vi "MCSControlPanel.vi"(4 "Register Map\nDefaults":refnum<vi>, 5 "StatusWord0x10Ref":refnum<vi>, 6 "Register Map\nRead Ref":refnum<vi>, 7 "NewRegMapReady":refnum<vi>, 8 "Last Command\nSent Ref":refnum<vi>, 9 "Stop Loop \nRef":refnum<vi>, 10 "error out":errorcluster, 11 "queue out":refnum<queue>) -> ()   [LabVIEW 2012]
panel:
  out "0x10 Status Word Readout":bool[][](array[boolean])
  in  "SYNC In \nVolt Threshold":u16
  out "word33":string
  in  "DIN In Volt \nThreshold":u16
  out "word32":string
  in  "DEMUX In Volt \nThreshold":u16
  out "word31":string
  in  "Power Mon Volt \nRef Threshold":u16
  out "word30":string
  out "wordB":string
  in  "Power Mon In 5 \nDEMUX Select":string(combo)
  in  "Power Mon In 4 \nDEMUX Select":string(combo)
  in  "Power Mon In 3 \nDEMUX Select":string(combo)
  in  "Power Mon In 2 \nDEMUX Select":string(combo)
  in  "Power Mon In 1 \nDEMUX Select":string(combo)
  in  "Power Mon In 0 \nDEMUX Select":string(combo)
  in  "Power Pulse\nReject Config":u16
  in  "Power Mon \nAcc Mode":string(combo)
  in  "Power Mon \nTest Mode":string(combo)
  in  "Power Mon Chan Enable   \n  11    10      9      8       7       6      5       4       3       2      1       0":bool[](array[boolean])
  out "word9":string
  in  "SoftDEMUX \nSelector Enable":bool
  in  "Sync Select 3B":string(combo)
  in  "Sync Select 2B":string(combo)
  in  "Sync Select 1B":string(combo)
  in  "Sync Select 0B":string(combo)
  in  "Sync Select 7":string(combo)
  in  "Sync Select 6":string(combo)
  in  "Sync Select 5":string(combo)
  in  "Sync Select 4":string(combo)
  in  "Sync Select 3A":string(combo)
  in  "Sync Select 2A":string(combo)
  in  "Sync Select 1A":string(combo)
  in  "Sync Select 0A":string(combo)
  in  "Sync Test\nMode Config":u32
  in  "Pulse Period\n(clock cycles -1)":u32
  in  "Channel DEMUX \nSelector":bool
  in  "Channel \nHold Order":bool
  in  "Channel \nTransfer Order":bool
  in  "Throttle Mode":string(combo)
  in  "Sync Test Mode Select":string(combo)
  in  "Data Input Test Mode":string(combo)
  out "Last Command Sent":string
  in  "Send Command, \nmanual entry":string
  in  "Send":bool
  in  "Reset Register Map to Defaults":bool
  in  "Sync Enable\n  2       1       0":bool[](array[boolean])
  in  "Channel Enable\n 11     10      9      8       7       6      5        4      3       2       1       0":bool[](array[boolean])
  in  "Reset Profile Accumulator  \n  11     10     9      8       7       6      5       4       3      2       1       0":bool[](array[boolean])
  in  "Counts Per Bin":u16
  in  "User Reset":bool
  in  "Number of Bins":u16
  in  "Profiles Per Histogram":u16
  in  "Time Reset":bool
  in  "Relative Time Step":u32
  in  "Demux Channel Enable\n  3       2       1      0":bool[](array[boolean])
  out "word0":string
  out "word1":string
  out "word2":string
  out "word3":string
  out "word4":string
  out "word5":string
  out "word6":string
  out "word7":string
  out "word8":string
  in  "DIN Polarity \n  7      6        5      4       3       2      1       0":bool[](array[boolean])
  in  "DIN Demux Polarity\n  3       2       1      0":bool[](array[boolean])
  in  "Sync Input Polarity\n  2       1       0":bool[](array[boolean])
  in  "PIN0 Pulse \nDurration Ave 2^N":u16
  out "wordA":string
  in  "PIN1 Pulse \nDurration Ave 2^N":u16
  in  "PIN2 Pulse \nDurration Ave 2^N":u16
  in  "PIN3 Pulse \nDurration Ave 2^N":u16
  in  "PIN4 Pulse \nDurration Ave 2^N":u16
  in  "PIN5 Pulse \nDurration Ave 2^N":u16
  # "word00"
  # "word30"
  # "valid range (0-65535)"
  # "word01"
  # "word02"
  # "word03"
  # "word04"
  # "word31"
  # "valid range (2-4096)"
  # "valid range (2-4096)"
  # "valid range (1-32,768)"
  # "valid range (0-65535)"
  # "word32"
  # "word05"
  # "valid range (0-65535)"
  # "word33"
  # "word06"
  # "valid range (0-65535)"
  # "valid range (0-256)"
  # "valid range (0-64)"
  # "word07"
  # "word08"
  # "word09"
  # "valid range (0-33,554,432)"
  # "valid range (0-256)"
  # "word0A"
  # "word0B"
  # "N=valid range (0-15)"
  # "N=valid range (0-15)"
  # "N=valid range (0-15)"
  # "N=valid range (0-15)"
  # "N=valid range (0-15)"
  # "N=valid range (0-15)"
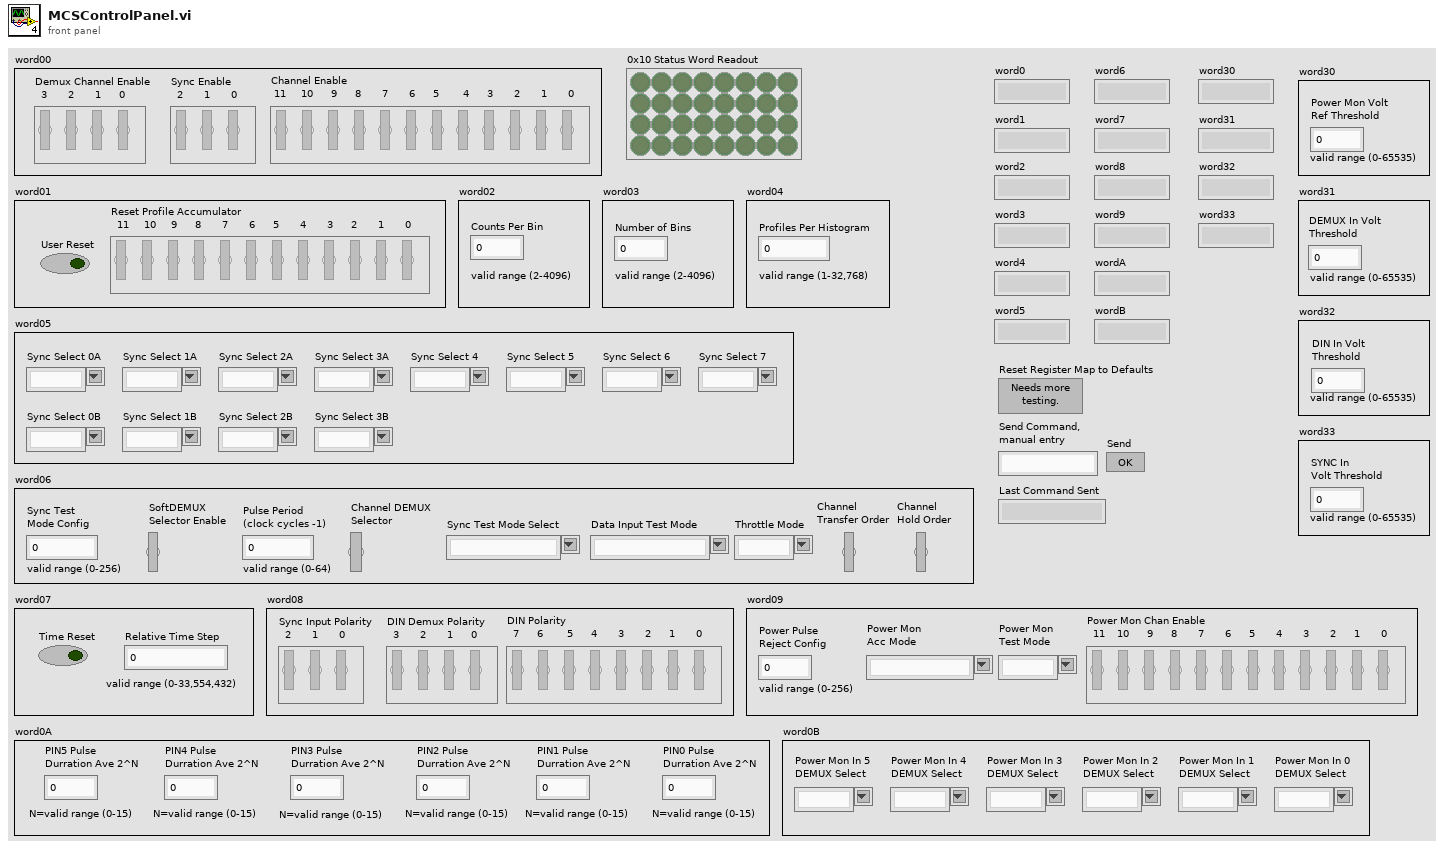
[diagram p1: front panel]
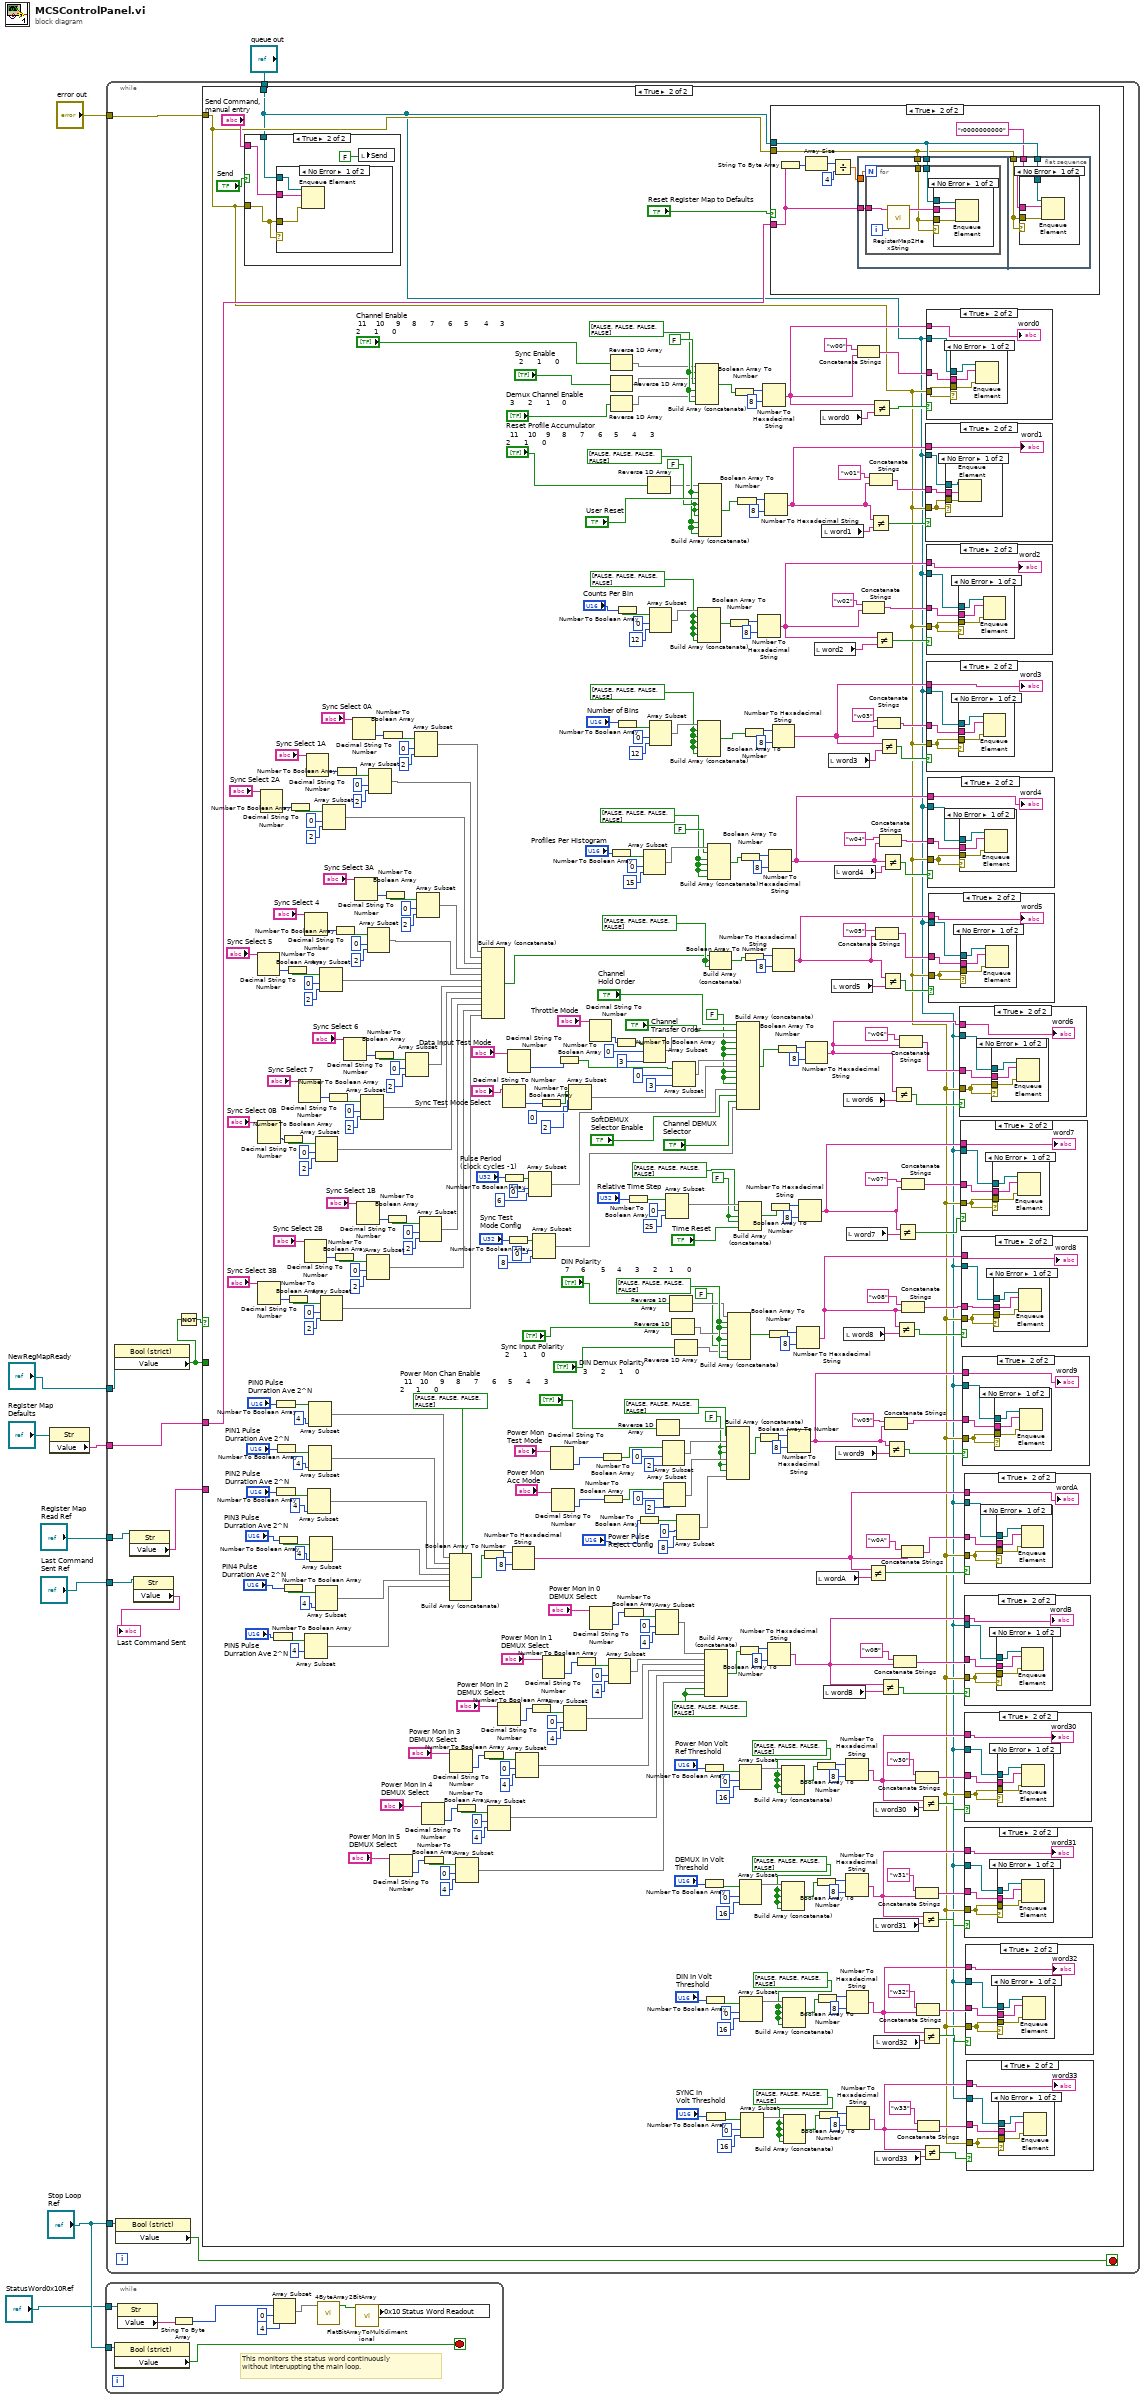
[diagram p0: block diagram]
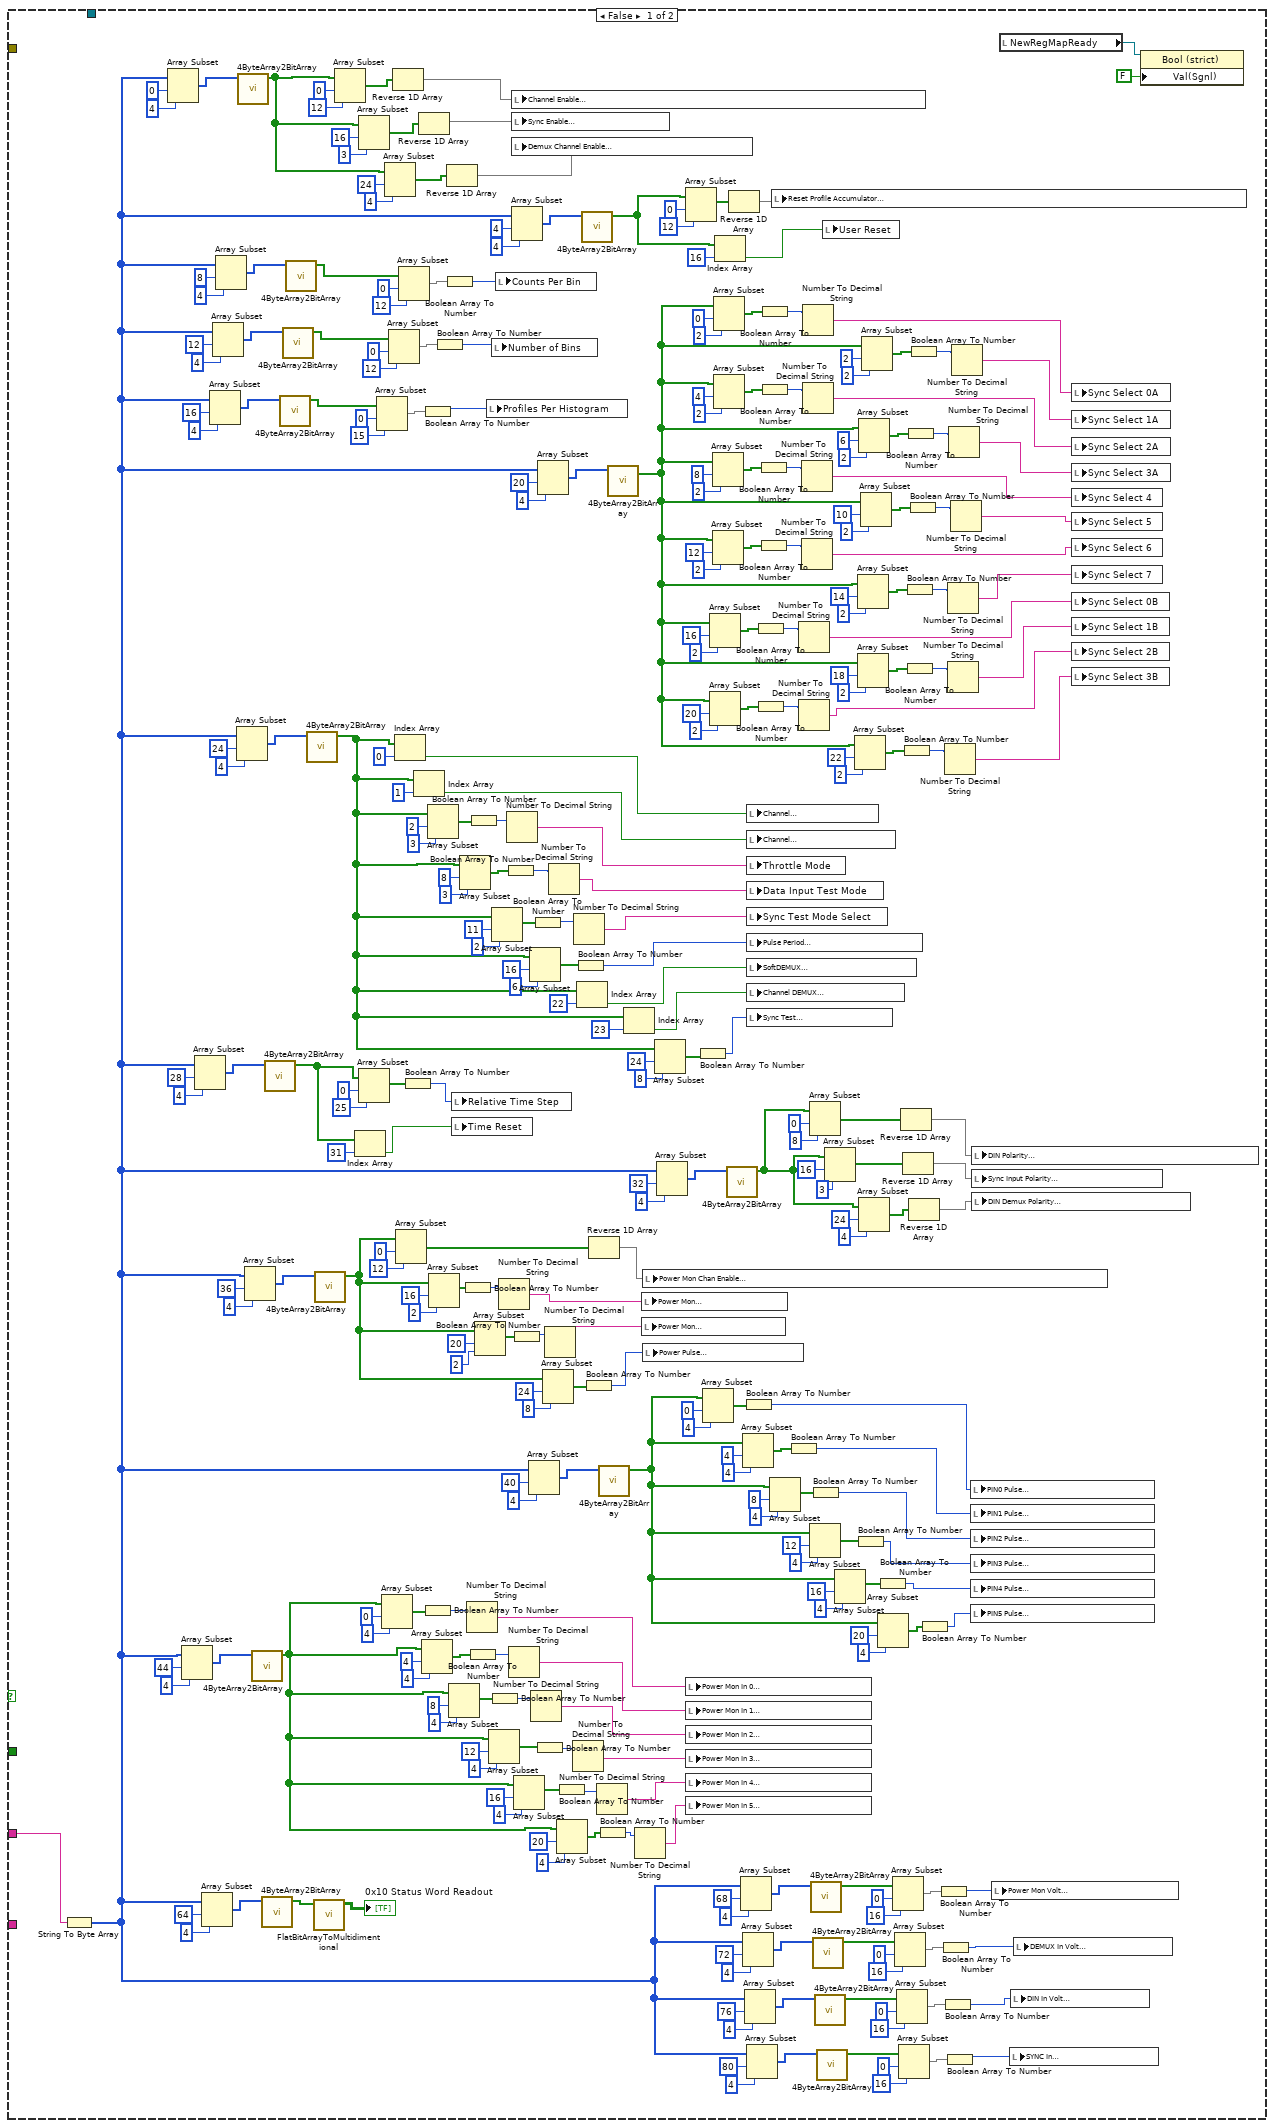
[diagram p2: hidden frame]
diagram:
  n1 = property class="Str"(reference="Register Map\nDefaults") -> ("Value"=w3:string)  [unwired: 1 in, 2 out]
  n2 = while {
    tunnel: "Stop Loop \nRef" -> [w14]
    tunnel: "StatusWord0x10Ref" -> [w11]
    stop <- w13 stop-if-true
    # "This monitors the status word continuously\nwithout interuppting the main loop."
    n3 = property class="Bool (strict)"(reference=w14) -> ("Value"=w13:bool)  [unwired: 1 in, 2 out]
    n4 = property class="Str"(reference=w11) -> ("Value"=w12:string)  [unwired: 1 in, 2 out]
    n5 = String To Byte Array(string=w12) -> (unsigned byte array=w17:u8[])
    n6 = Array Subset(array=w17, index=0, length=4) -> (w16:u8[])
    n7 = call "4ByteArray2BitArray.vi"("array"=w16) -> ("Array"=w15:bool[])  [unwired: 10 in]
    n8 = call "FlatBitArrayToMultidimentional.vi"("Array in"=w15) -> ("Array out"=w10:bool[][])  [unwired: 10 in]
    n9 = local write "0x10 Status Word Readout"(w10) -> ()
  }
  n10 = while {
    tunnel: "queue out" -> [w31]
    tunnel: "error out" -> [w30]
    tunnel: "Stop Loop \nRef" -> [w29]
    tunnel: "Last Command\nSent Ref" -> [w25]
    tunnel: "Register Map\nRead Ref" -> [w26]
    tunnel: w3 -> [w22]
    tunnel: "NewRegMapReady" -> [w23]
    stop <- w28 stop-if-true
    n11 = property class="Bool (strict)"(reference=w23) -> ("Value"=w20:bool)  [unwired: 1 in, 2 out]
    n12 = property class="Bool (strict)"(reference=w29) -> ("Value"=w28:bool)  [unwired: 1 in, 2 out]
    n13 = property class="Str"(reference=w26) -> ("Value"=w24:string)  [unwired: 1 in, 2 out]
    n14 = property class="Str"(reference=w25) -> ("Value"=→"Last Command Sent":string)  [unwired: 1 in, 2 out]
    n15 = Not(x=w20) -> (.not. x?=w21:bool)
    n16 = case shown="True" w21 {
      tunnel: w31 -> [_ w338]
      tunnel: w30 -> [_ w339]
      tunnel: w24 -> [_ _]
      tunnel: w22 -> [w54 w514]
      tunnel: w20 -> [_ _]
      frame False {
        n17 = String To Byte Array(string=w54) -> (unsigned byte array=w51:u8[])
        n18 = Array Subset(array=w51, index=0, length=4) -> (w300:u8[])
        n19 = Array Subset(array=w51, index=44, length=4) -> (w118:u8[])
        n20 = Array Subset(array=w51, index=28, length=4) -> (w306:u8[])
        n21 = Array Subset(array=w51, index=64, length=4) -> (w50:u8[])
        n22 = Array Subset(array=w51, index=16, length=4) -> (w315:u8[])
        n23 = Array Subset(array=w51, index=12, length=4) -> (w318:u8[])
        n24 = Array Subset(array=w51, index=8, length=4) -> (w321:u8[])
        n25 = Array Subset(array=w51, index=24, length=4) -> (w309:u8[])
        n26 = call "4ByteArray2BitArray.vi"("array"=w300) -> ("Array"=w146:bool[])  [unwired: 10 in]
        n27 = Array Subset(array=w51, index=36, length=4) -> (w140:u8[])
        n28 = call "4ByteArray2BitArray.vi"("array"=w118) -> ("Array"=w99:bool[])  [unwired: 10 in]
        n29 = call "4ByteArray2BitArray.vi"("array"=w50) -> ("Array"=w33:bool[])  [unwired: 10 in]
        n30 = call "4ByteArray2BitArray.vi"("array"=w306) -> ("Array"=w265:bool[])  [unwired: 10 in]
        n31 = call "4ByteArray2BitArray.vi"("array"=w315) -> ("Array"=w167:bool[])  [unwired: 10 in]
        n32 = call "4ByteArray2BitArray.vi"("array"=w318) -> ("Array"=w162:bool[])  [unwired: 10 in]
        n33 = call "4ByteArray2BitArray.vi"("array"=w321) -> ("Array"=w157:bool[])  [unwired: 10 in]
        n34 = call "4ByteArray2BitArray.vi"("array"=w309) -> ("Array"=w145:bool[])  [unwired: 10 in]
        n35 = call "FlatBitArrayToMultidimentional.vi"("Array in"=w33) -> ("Array out"=→"0x10 Status Word Readout":bool[][])  [unwired: 10 in]
        n36 = call "4ByteArray2BitArray.vi"("array"=w140) -> ("Array"=w127:bool[])  [unwired: 10 in]
        n37 = Array Subset(array=w146, index=0, length=12) -> (w48:bool[])
        n38 = Index Array(array=w265, index=31) -> (element=w263:bool)
        n39 = Array Subset(array=w146, index=16, length=3) -> (w46:bool[])
        n40 = Array Subset(array=w265, index=0, length=25) -> (w261:bool[])
        n41 = Array Subset(array=w167, index=0, length=15) -> (w168:bool[])
        n42 = Array Subset(array=w99, index=0, length=4) -> (w104:bool[])
        n43 = Array Subset(array=w146, index=24, length=4) -> (w44:bool[])
        n44 = Array Subset(array=w162, index=0, length=12) -> (w163:bool[])
        n45 = Reverse 1D Array(array=w48) -> (reversed array=w49:bool[])
        n46 = Index Array(array=w145, index=0) -> (element=w243:bool)
        n47 = Array Subset(array=w127, index=0, length=12) -> (w34:bool[])
        n48 = Array Subset(array=w157, index=0, length=12) -> (w158:bool[])
        n49 = Boolean Array To Number(Boolean array=w261) -> (number=w262:u32)
        n50 = Index Array(array=w145, index=1) -> (element=w242:bool)
        n51 = Reverse 1D Array(array=w46) -> (reversed array=w47:bool[])
        n52 = Array Subset(array=w99, index=4, length=4) -> (w105:bool[])
        n53 = Boolean Array To Number(Boolean array=w168) -> (number=w166:u32)
        n54 = Boolean Array To Number(Boolean array=w104) -> (number=w98:u32)
        n55 = Array Subset(array=w145, index=2, length=3) -> (w249:bool[])
        n56 = Array Subset(array=w127, index=16, length=2) -> (w136:bool[])
        n57 = Boolean Array To Number(Boolean array=w163) -> (number=w161:u32)
        n58 = Boolean Array To Number(Boolean array=w158) -> (number=w156:u32)
        n59 = Reverse 1D Array(array=w44) -> (reversed array=w45:bool[])
        n60 = Array Subset(array=w99, index=8, length=4) -> (w103:bool[])
        n61 = local write "Relative Time Step"(w262) -> ()
        n62 = local write "Time Reset"(w263) -> ()
        n63 = Array Subset(array=w145, index=8, length=3) -> (w250:bool[])
        n64 = Boolean Array To Number(Boolean array=w136) -> (number=w135:u32)
        n65 = Number To Decimal String(number=w98) -> (decimal integer string=w87:string)  [unwired: 1 in]
        n66 = Boolean Array To Number(Boolean array=w105) -> (number=w97:u32)
        n67 = Boolean Array To Number(Boolean array=w249) -> (number=w241:u32)
        n68 = Array Subset(array=w127, index=20, length=2) -> (w132:bool[])
        n69 = local write "Profiles Per Histogram"(w166) -> ()
        n70 = Array Subset(array=w99, index=12, length=4) -> (w102:bool[])
        n71 = Boolean Array To Number(Boolean array=w103) -> (number=w96:u32)
        n72 = local write "Number of Bins"(w161) -> ()
        n73 = Array Subset(array=w145, index=11, length=2) -> (w248:bool[])
        n74 = local write "Counts Per Bin"(w156) -> ()
        n75 = Number To Decimal String(number=w135) -> (decimal integer string=w134:string)  [unwired: 1 in]
        n76 = Boolean Array To Number(Boolean array=w250) -> (number=w239:u32)
        n77 = Number To Decimal String(number=w241) -> (decimal integer string=w240:string)  [unwired: 1 in]
        n78 = Number To Decimal String(number=w97) -> (decimal integer string=w88:string)  [unwired: 1 in]
        n79 = local write "Channel Enable\n 11     10      9      8       7       6      5        4      3       2       1       0"(w49) -> ()
        n80 = local write "Sync Enable\n  2       1       0"(w47) -> ()
        n81 = local write "Demux Channel Enable\n  3       2       1      0"(w45) -> ()
        n82 = Array Subset(array=w51, index=4, length=4) -> (w324:u8[])
        n83 = Boolean Array To Number(Boolean array=w132) -> (number=w131:u32)
        n84 = Array Subset(array=w99, index=16, length=4) -> (w101:bool[])
        n85 = Array Subset(array=w51, index=40, length=4) -> (w327:u8[])
        n86 = Array Subset(array=w145, index=16, length=6) -> (w247:bool[])
        n87 = Number To Decimal String(number=w96) -> (decimal integer string=w89:string)  [unwired: 1 in]
        n88 = Boolean Array To Number(Boolean array=w248) -> (number=w237:u32)
        n89 = Boolean Array To Number(Boolean array=w102) -> (number=w94:u32)
        n90 = Array Subset(array=w51, index=20, length=4) -> (w312:u8[])
        n91 = Array Subset(array=w127, index=24, length=8) -> (w128:bool[])
        n92 = Number To Decimal String(number=w131) -> (decimal integer string=w130:string)  [unwired: 1 in]
        n93 = Number To Decimal String(number=w239) -> (decimal integer string=w238:string)  [unwired: 1 in]
        n94 = Boolean Array To Number(Boolean array=w101) -> (number=w95:u32)
        n95 = Array Subset(array=w99, index=20, length=4) -> (w100:bool[])
        n96 = Number To Decimal String(number=w94) -> (decimal integer string=w90:string)  [unwired: 1 in]
        n97 = Number To Decimal String(number=w237) -> (decimal integer string=w236:string)  [unwired: 1 in]
        n98 = Boolean Array To Number(Boolean array=w247) -> (number=w233:u32)
        n99 = Index Array(array=w145, index=22) -> (element=w143:bool)
        n100 = call "4ByteArray2BitArray.vi"("array"=w324) -> ("Array"=w152:bool[])  [unwired: 10 in]
        n101 = Boolean Array To Number(Boolean array=w128) -> (number=w126:u32)
        n102 = Reverse 1D Array(array=w34) -> (reversed array=w35:bool[])
        n103 = Number To Decimal String(number=w95) -> (decimal integer string=w91:string)  [unwired: 1 in]
        n104 = Boolean Array To Number(Boolean array=w100) -> (number=w93:u32)
        n105 = call "4ByteArray2BitArray.vi"("array"=w327) -> ("Array"=w287:bool[])  [unwired: 10 in]
        n106 = call "4ByteArray2BitArray.vi"("array"=w312) -> ("Array"=w183:bool[])  [unwired: 10 in]
        n107 = Index Array(array=w145, index=23) -> (element=w234:bool)
        n108 = Number To Decimal String(number=w93) -> (decimal integer string=w92:string)  [unwired: 1 in]
        n109 = local write "Power Mon \nTest Mode"(w134) -> ()
        n110 = local write "Power Mon \nAcc Mode"(w130) -> ()
        n111 = local write "Power Mon Chan Enable   \n  11    10      9      8       7       6      5       4       3       2      1       0"(w35) -> ()
        n112 = local write "Power Pulse\nReject Config"(w126) -> ()
        n113 = Array Subset(array=w145, index=24, length=8) -> (w246:bool[])
        n114 = Array Subset(array=w51, index=32, length=4) -> (w303:u8[])
        n115 = Array Subset(array=w152, index=0, length=12) -> (w42:bool[])
        n116 = local write "Power Mon In 0 \nDEMUX Select"(w87) -> ()
        n117 = local write "Power Mon In 1 \nDEMUX Select"(w88) -> ()
        n118 = local write "Power Mon In 2 \nDEMUX Select"(w89) -> ()
        n119 = local write "Power Mon In 3 \nDEMUX Select"(w90) -> ()
        n120 = local write "Power Mon In 4 \nDEMUX Select"(w91) -> ()
        n121 = local write "Power Mon In 5 \nDEMUX Select"(w92) -> ()
        n122 = Boolean Array To Number(Boolean array=w246) -> (number=w232:u32)
        n123 = Array Subset(array=w287, index=0, length=4) -> (w284:bool[])
        n124 = Array Subset(array=w183, index=16, length=2) -> (w197:bool[])
        n125 = Array Subset(array=w183, index=20, length=2) -> (w189:bool[])
        n126 = Array Subset(array=w183, index=8, length=2) -> (w213:bool[])
        n127 = Array Subset(array=w183, index=12, length=2) -> (w205:bool[])
        n128 = Array Subset(array=w183, index=0, length=2) -> (w229:bool[])
        n129 = Array Subset(array=w183, index=4, length=2) -> (w221:bool[])
        n130 = Index Array(array=w152, index=16) -> (element=w151:bool)
        n131 = call "4ByteArray2BitArray.vi"("array"=w303) -> ("Array"=w268:bool[])  [unwired: 10 in]
        n132 = Reverse 1D Array(array=w42) -> (reversed array=w43:bool[])
        n133 = Array Subset(array=w51, index=68, length=4) -> (w84:u8[])
        n134 = Array Subset(array=w287, index=4, length=4) -> (w286:bool[])
        n135 = Array Subset(array=w51, index=72, length=4) -> (w77:u8[])
        n136 = Boolean Array To Number(Boolean array=w284) -> (number=w283:u32)
        n137 = Array Subset(array=w51, index=76, length=4) -> (w70:u8[])
        n138 = local write "Channel \nHold Order"(w243) -> ()
        n139 = local write "Channel \nTransfer Order"(w242) -> ()
        n140 = local write "Throttle Mode"(w240) -> ()
        n141 = local write "Data Input Test Mode"(w238) -> ()
        n142 = local write "Sync Test Mode Select"(w236) -> ()
        n143 = local write "Pulse Period\n(clock cycles -1)"(w233) -> ()
        n144 = local write "SoftDEMUX \nSelector Enable"(w143) -> ()
        n145 = local write "Channel DEMUX \nSelector"(w234) -> ()
        n146 = local write "Sync Test\nMode Config"(w232) -> ()
        n147 = Array Subset(array=w51, index=80, length=4) -> (w63:u8[])
        n148 = Boolean Array To Number(Boolean array=w197) -> (number=w196:u32)
        n149 = Boolean Array To Number(Boolean array=w189) -> (number=w188:u32)
        n150 = Boolean Array To Number(Boolean array=w213) -> (number=w212:u32)
        n151 = Boolean Array To Number(Boolean array=w205) -> (number=w204:u32)
        n152 = Boolean Array To Number(Boolean array=w229) -> (number=w228:u32)
        n153 = Boolean Array To Number(Boolean array=w221) -> (number=w220:u32)
        n154 = Array Subset(array=w287, index=8, length=4) -> (w281:bool[])
        n155 = local write "Reset Profile Accumulator  \n  11     10     9      8       7       6      5       4       3      2       1       0"(w43) -> ()
        n156 = Boolean Array To Number(Boolean array=w286) -> (number=w285:u32)
        n157 = Number To Decimal String(number=w196) -> (decimal integer string=w174:string)  [unwired: 1 in]
        n158 = Number To Decimal String(number=w188) -> (decimal integer string=w172:string)  [unwired: 1 in]
        n159 = Number To Decimal String(number=w212) -> (decimal integer string=w178:string)  [unwired: 1 in]
        n160 = Number To Decimal String(number=w204) -> (decimal integer string=w176:string)  [unwired: 1 in]
        n161 = Number To Decimal String(number=w228) -> (decimal integer string=w182:string)  [unwired: 1 in]
        n162 = Number To Decimal String(number=w220) -> (decimal integer string=w180:string)  [unwired: 1 in]
        n163 = Array Subset(array=w268, index=0, length=8) -> (w36:bool[])
        n164 = Array Subset(array=w287, index=12, length=4) -> (w280:bool[])
        n165 = Boolean Array To Number(Boolean array=w281) -> (number=w282:u32)
        n166 = call "4ByteArray2BitArray.vi"("array"=w84) -> ("Array"=w80:bool[])  [unwired: 10 in]
        n167 = call "4ByteArray2BitArray.vi"("array"=w77) -> ("Array"=w73:bool[])  [unwired: 10 in]
        n168 = call "4ByteArray2BitArray.vi"("array"=w70) -> ("Array"=w66:bool[])  [unwired: 10 in]
        n169 = call "4ByteArray2BitArray.vi"("array"=w63) -> ("Array"=w59:bool[])  [unwired: 10 in]
        n170 = local write "User Reset"(w151) -> ()
        n171 = Array Subset(array=w268, index=16, length=3) -> (w37:bool[])
        n172 = Array Subset(array=w287, index=16, length=4) -> (w279:bool[])
        n173 = Array Subset(array=w183, index=22, length=2) -> (w185:bool[])
        n174 = Boolean Array To Number(Boolean array=w280) -> (number=w275:u32)
        n175 = Array Subset(array=w183, index=14, length=2) -> (w201:bool[])
        n176 = Array Subset(array=w183, index=18, length=2) -> (w193:bool[])
        n177 = Array Subset(array=w183, index=6, length=2) -> (w217:bool[])
        n178 = Array Subset(array=w268, index=24, length=4) -> (w38:bool[])
        n179 = Array Subset(array=w183, index=10, length=2) -> (w209:bool[])
        n180 = Array Subset(array=w183, index=2, length=2) -> (w225:bool[])
        n181 = Boolean Array To Number(Boolean array=w279) -> (number=w276:u32)
        n182 = Array Subset(array=w287, index=20, length=4) -> (w278:bool[])
        n183 = Array Subset(array=w80, index=0, length=16) -> (w81:bool[])
        n184 = Array Subset(array=w73, index=0, length=16) -> (w74:bool[])
        n185 = Array Subset(array=w66, index=0, length=16) -> (w67:bool[])
        n186 = Array Subset(array=w59, index=0, length=16) -> (w60:bool[])
        n187 = Reverse 1D Array(array=w36) -> (reversed array=w41:bool[])
        n188 = Boolean Array To Number(Boolean array=w185) -> (number=w184:u32)
        n189 = Reverse 1D Array(array=w37) -> (reversed array=w40:bool[])
        n190 = Boolean Array To Number(Boolean array=w201) -> (number=w200:u32)
        n191 = Boolean Array To Number(Boolean array=w193) -> (number=w192:u32)
        n192 = Boolean Array To Number(Boolean array=w217) -> (number=w216:u32)
        n193 = Boolean Array To Number(Boolean array=w209) -> (number=w208:u32)
        n194 = Boolean Array To Number(Boolean array=w225) -> (number=w224:u32)
        n195 = Reverse 1D Array(array=w38) -> (reversed array=w39:bool[])
        n196 = Boolean Array To Number(Boolean array=w278) -> (number=w277:u32)
        n197 = Boolean Array To Number(Boolean array=w81) -> (number=w58:u32)
        n198 = Boolean Array To Number(Boolean array=w74) -> (number=w57:u32)
        n199 = Boolean Array To Number(Boolean array=w67) -> (number=w56:u32)
        n200 = Number To Decimal String(number=w184) -> (decimal integer string=w171:string)  [unwired: 1 in]
        n201 = Boolean Array To Number(Boolean array=w60) -> (number=w55:u32)
        n202 = Number To Decimal String(number=w200) -> (decimal integer string=w175:string)  [unwired: 1 in]
        n203 = Number To Decimal String(number=w192) -> (decimal integer string=w173:string)  [unwired: 1 in]
        n204 = Number To Decimal String(number=w216) -> (decimal integer string=w179:string)  [unwired: 1 in]
        n205 = Number To Decimal String(number=w208) -> (decimal integer string=w177:string)  [unwired: 1 in]
        n206 = Number To Decimal String(number=w224) -> (decimal integer string=w181:string)  [unwired: 1 in]
        n207 = local write "PIN0 Pulse \nDurration Ave 2^N"(w283) -> ()
        n208 = local write "PIN1 Pulse \nDurration Ave 2^N"(w285) -> ()
        n209 = local write "PIN2 Pulse \nDurration Ave 2^N"(w282) -> ()
        n210 = local write "PIN3 Pulse \nDurration Ave 2^N"(w275) -> ()
        n211 = local write "PIN4 Pulse \nDurration Ave 2^N"(w276) -> ()
        n212 = local write "PIN5 Pulse \nDurration Ave 2^N"(w277) -> ()
        n213 = local write "DIN Polarity \n  7      6        5      4       3       2      1       0"(w41) -> ()
        n214 = local write "Sync Input Polarity\n  2       1       0"(w40) -> ()
        n215 = local write "DIN Demux Polarity\n  3       2       1      0"(w39) -> ()
        n216 = local write "Power Mon Volt \nRef Threshold"(w58) -> ()
        n217 = local read "NewRegMapReady"() -> (w122:refnum<vi>)
        n218 = local write "SYNC In \nVolt Threshold"(w55) -> ()
        n219 = local write "DIN In Volt \nThreshold"(w56) -> ()
        n220 = local write "DEMUX In Volt \nThreshold"(w57) -> ()
        n221 = local write "Sync Select 0A"(w182) -> ()
        n222 = local write "Sync Select 1A"(w181) -> ()
        n223 = local write "Sync Select 2A"(w180) -> ()
        n224 = local write "Sync Select 3A"(w179) -> ()
        n225 = local write "Sync Select 4"(w178) -> ()
        n226 = local write "Sync Select 5"(w177) -> ()
        n227 = local write "Sync Select 6"(w176) -> ()
        n228 = local write "Sync Select 7"(w175) -> ()
        n229 = local write "Sync Select 0B"(w174) -> ()
        n230 = local write "Sync Select 1B"(w173) -> ()
        n231 = local write "Sync Select 2B"(w172) -> ()
        n232 = local write "Sync Select 3B"(w171) -> ()
        n233 = property class="Bool (strict)"(reference=w122, "Val(Sgnl)"=FALSE ("Value (Signaling)")) -> ()  [unwired: 1 in, 2 out]
      }
      frame True {
        w340 = bool[] [FALSE, FALSE, FALSE, FALSE] ("appended array")
        w354 = bool[] [FALSE, FALSE, FALSE, FALSE] ("appended array")
        w368 = bool[] [FALSE, FALSE, FALSE, FALSE] ("appended array")
        w382 = bool[] [FALSE, FALSE, FALSE, FALSE] ("appended array")
        w443 = bool[] [FALSE, FALSE, FALSE, FALSE] ("appended array")
        w333 = FALSE ("Read Register")
        w666 = bool[] [FALSE, FALSE, FALSE, FALSE] ("appended array")
        w690 = bool[] [FALSE, FALSE, FALSE, FALSE] ("appended array")
        w692 = FALSE ("Read Register")
        w625 = FALSE ("Read Register")
        w697 = bool[] [FALSE, FALSE, FALSE, FALSE] ("appended array")
        w546 = bool[] [FALSE, FALSE, FALSE, FALSE] ("appended array")
        w695 = bool[] [FALSE, FALSE, FALSE, FALSE] ("appended array")
        w696 = bool[] [FALSE, FALSE, FALSE, FALSE] ("appended array")
        w710 = FALSE ("Read Register")
        w709 = bool[] [FALSE, FALSE, FALSE, FALSE] ("appended array")
        w712 = bool[] [FALSE, FALSE, FALSE, FALSE] ("appended array")
        n234 = case shown="True" "Send" {
          tunnel: "Send Command, \nmanual entry" -> [_ w869]
          tunnel: w338 -> [_ w868]
          tunnel: w339 -> [_ w866]
          frame False {
          }
          frame True {
            n235 = case shown="No Error" w866 {
              tunnel: w869 -> [w872 _]
              tunnel: w866 -> [w871 _]
              tunnel: w868 -> [w870 _]
              frame No Error {
                n236 = Enqueue Element(queue=w870, element=w872, error in (no error)=w871) -> ()  [unwired: 1 in, 3 out]
              }
              frame Error {
              }
            }
            n237 = local write "Send"(FALSE ("Send")) -> ()
          }
        }
        n238 = Decimal String To Number(string="Sync Select 5") -> (number=w590:i32)  [unwired: 2 in, 1 out]
        n239 = Decimal String To Number(string="Sync Select 0B") -> (number=w575:i32)  [unwired: 2 in, 1 out]
        n240 = Decimal String To Number(string="Sync Select 3B") -> (number=w560:i32)  [unwired: 2 in, 1 out]
        n241 = Decimal String To Number(string="Sync Select 2A") -> (number=w605:i32)  [unwired: 2 in, 1 out]
        n242 = Number To Boolean Array(number="PIN5 Pulse \nDurration Ave 2^N") -> (Boolean array=w682:bool[])
        n243 = Number To Boolean Array(number="PIN0 Pulse \nDurration Ave 2^N") -> (Boolean array=w688:bool[])
        n244 = Number To Boolean Array(number="PIN2 Pulse \nDurration Ave 2^N") -> (Boolean array=w678:bool[])
        n245 = Number To Boolean Array(number="PIN1 Pulse \nDurration Ave 2^N") -> (Boolean array=w686:bool[])
        n246 = Number To Boolean Array(number="PIN3 Pulse \nDurration Ave 2^N") -> (Boolean array=w680:bool[])
        n247 = Number To Boolean Array(number=w575) -> (Boolean array=w577:bool[])
        n248 = Number To Boolean Array(number="PIN4 Pulse \nDurration Ave 2^N") -> (Boolean array=w684:bool[])
        n249 = Number To Boolean Array(number=w590) -> (Boolean array=w592:bool[])
        n250 = Number To Boolean Array(number=w560) -> (Boolean array=w562:bool[])
        n251 = Number To Boolean Array(number=w605) -> (Boolean array=w607:bool[])
        n252 = Decimal String To Number(string="Sync Select 7") -> (number=w580:i32)  [unwired: 2 in, 1 out]
        n253 = Decimal String To Number(string="Sync Select 2B") -> (number=w565:i32)  [unwired: 2 in, 1 out]
        n254 = Decimal String To Number(string="Sync Select 4") -> (number=w595:i32)  [unwired: 2 in, 1 out]
        n255 = Array Subset(array=w682, length=4) -> (w667:bool[])  [unwired: 1 in]
        n256 = Decimal String To Number(string="Sync Select 1A") -> (number=w610:i32)  [unwired: 2 in, 1 out]
        n257 = Array Subset(array=w678, length=4) -> (w670:bool[])  [unwired: 1 in]
        n258 = Array Subset(array=w688, length=4) -> (w672:bool[])  [unwired: 1 in]
        n259 = Array Subset(array=w686, length=4) -> (w671:bool[])  [unwired: 1 in]
        n260 = Array Subset(array=w680, length=4) -> (w669:bool[])  [unwired: 1 in]
        n261 = Array Subset(array=w577, index=0, length=2) -> (w550:bool[])
        n262 = Array Subset(array=w684, length=4) -> (w668:bool[])  [unwired: 1 in]
        n263 = Array Subset(array=w592, index=0, length=2) -> (w554:bool[])
        n264 = Array Subset(array=w562, index=0, length=2) -> (w553:bool[])
        n265 = Array Subset(array=w607, index=0, length=2) -> (w557:bool[])
        n266 = Number To Boolean Array(number=w580) -> (Boolean array=w582:bool[])
        n267 = Number To Boolean Array(number=w565) -> (Boolean array=w567:bool[])
        n268 = Number To Boolean Array(number=w595) -> (Boolean array=w597:bool[])
        n269 = Number To Boolean Array(number=w610) -> (Boolean array=w612:bool[])
        n270 = Decimal String To Number(string="Sync Select 6") -> (number=w585:i32)  [unwired: 2 in, 1 out]
        n271 = Decimal String To Number(string="Sync Select 0A") -> (number=w615:i32)  [unwired: 2 in, 1 out]
        n272 = Decimal String To Number(string="Sync Select 3A") -> (number=w600:i32)  [unwired: 2 in, 1 out]
        n273 = Decimal String To Number(string="Sync Select 1B") -> (number=w570:i32)  [unwired: 2 in, 1 out]
        n274 = Array Subset(array=w582, index=0, length=2) -> (w549:bool[])
        n275 = Array Subset(array=w567, index=0, length=2) -> (w552:bool[])
        n276 = Array Subset(array=w597, index=0, length=2) -> (w555:bool[])
        n277 = Array Subset(array=w612, index=0, length=2) -> (w558:bool[])
        n278 = Number To Boolean Array(number=w585) -> (Boolean array=w587:bool[])
        n279 = Number To Boolean Array(number=w615) -> (Boolean array=w617:bool[])
        n280 = Number To Boolean Array(number=w600) -> (Boolean array=w602:bool[])
        n281 = Number To Boolean Array(number=w570) -> (Boolean array=w572:bool[])
        n282 = Decimal String To Number(string="Power Mon In 5 \nDEMUX Select") -> (number=w446:i32)  [unwired: 2 in, 1 out]
        n283 = Array Subset(array=w587, index=0, length=2) -> (w548:bool[])
        n284 = Array Subset(array=w617, index=0, length=2) -> (w559:bool[])
        n285 = Array Subset(array=w602, index=0, length=2) -> (w556:bool[])
        n286 = Array Subset(array=w572, index=0, length=2) -> (w551:bool[])
        n287 = Decimal String To Number(string="Power Mon In 4 \nDEMUX Select") -> (number=w456:i32)  [unwired: 2 in, 1 out]
        n288 = Number To Boolean Array(number=w446) -> (Boolean array=w447:bool[])
        n289 = Build Array (concatenate)(w672, w671, w670, w669, w668, w667, w666, w666) -> (w515:bool[])
        n290 = Decimal String To Number(string="Power Mon In 3 \nDEMUX Select") -> (number=w461:i32)  [unwired: 2 in, 1 out]
        n291 = Number To Boolean Array(number=w456) -> (Boolean array=w457:bool[])
        n292 = Array Subset(array=w447, index=0, length=4) -> (w444:bool[])
        n293 = Build Array (concatenate)(w559, w558, w557, w556, w555, w554, w548, w549, w550, w551, w552, w553) -> (w647:bool[])
        n294 = Boolean Array To Number(Boolean array=w515) -> (number=w525:u32)
        n295 = Number To Boolean Array(number=w461) -> (Boolean array=w462:bool[])
        n296 = Array Subset(array=w457, index=0, length=4) -> (w450:bool[])
        n297 = Decimal String To Number(string="Power Mon In 2 \nDEMUX Select") -> (number=w466:i32)  [unwired: 2 in, 1 out]
        n298 = Decimal String To Number(string="Sync Test Mode Select") -> (number=w641:i32)  [unwired: 2 in, 1 out]
        n299 = Number To Boolean Array(number="Pulse Period\n(clock cycles -1)") -> (Boolean array=w634:bool[])
        n300 = Number To Boolean Array(number="Sync Test\nMode Config") -> (Boolean array=w624:bool[])
        n301 = Decimal String To Number(string="Data Input Test Mode") -> (number=w642:i32)  [unwired: 2 in, 1 out]
        n302 = Number To Hexadecimal String(1:i16 8 ("width (-)"), 2:w525) -> (0:w441:string)
        n303 = Array Subset(array=w462, index=0, length=4) -> (w451:bool[])
        n304 = Array Subset(array=w634, index=0, length=6) -> (w512:bool[])
        n305 = Number To Boolean Array(number=w466) -> (Boolean array=w467:bool[])
        n306 = Array Subset(array=w624, index=0, length=8) -> (w513:bool[])
        n307 = Number To Boolean Array(number=w641) -> (Boolean array=w635:bool[])
        n308 = Decimal String To Number(string="Power Mon In 1 \nDEMUX Select") -> (number=w471:i32)  [unwired: 2 in, 1 out]
        n309 = Decimal String To Number(string="Power Mon \nTest Mode") -> (number=w501:i32)  [unwired: 2 in, 1 out]
        n310 = Decimal String To Number(string="Power Mon \nAcc Mode") -> (number=w496:i32)  [unwired: 2 in, 1 out]
        n311 = Number To Boolean Array(number=w642) -> (Boolean array=w636:bool[])
        n312 = Array Subset(array=w467, index=0, length=4) -> (w452:bool[])
        n313 = Array Subset(array=w635, index=0, length=2) -> (w626:bool[])
        n314 = Number To Boolean Array(number=w471) -> (Boolean array=w472:bool[])
        n315 = Decimal String To Number(string="Throttle Mode") -> (number=w645:i32)  [unwired: 2 in, 1 out]
        n316 = Decimal String To Number(string="Power Mon In 0 \nDEMUX Select") -> (number=w476:i32)  [unwired: 2 in, 1 out]
        n317 = Number To Boolean Array(number=w501) -> (Boolean array=w500:bool[])
        n318 = Number To Boolean Array(number=w496) -> (Boolean array=w495:bool[])
        n319 = Array Subset(array=w472, index=0, length=4) -> (w453:bool[])
        n320 = Reverse 1D Array(array="Channel Enable\n 11     10      9      8       7       6      5        4      3       2       1       0") -> (reversed array=w399:bool[])
        n321 = Reverse 1D Array(array="Sync Enable\n  2       1       0") -> (reversed array=w400:bool[])
        n322 = Reverse 1D Array(array="Demux Channel Enable\n  3       2       1      0") -> (reversed array=w401:bool[])
        n323 = Number To Boolean Array(number="Profiles Per Histogram") -> (Boolean array=w700:bool[])
        n324 = Number To Boolean Array(number=w645) -> (Boolean array=w719:bool[])
        n325 = Number To Boolean Array(number="Counts Per Bin") -> (Boolean array=w722:bool[])
        n326 = Number To Boolean Array(number="Number of Bins") -> (Boolean array=w705:bool[])
        n327 = Number To Boolean Array(number=w476) -> (Boolean array=w477:bool[])
        n328 = Number To Boolean Array(number="Relative Time Step") -> (Boolean array=w716:bool[])
        n329 = Number To Boolean Array(number="Power Pulse\nReject Config") -> (Boolean array=w490:bool[])
        n330 = Array Subset(array=w700, index=0, length=15) -> (w699:bool[])
        n331 = Array Subset(array=w719, index=0, length=3) -> (w630:bool[])
        n332 = Reverse 1D Array(array="Reset Profile Accumulator  \n  11     10     9      8       7       6      5       4       3      2       1       0") -> (reversed array=w402:bool[])
        n333 = Array Subset(array=w722, index=0, length=12) -> (w708:bool[])
        n334 = Array Subset(array=w705, index=0, length=12) -> (w704:bool[])
        n335 = Array Subset(array=w477, index=0, length=4) -> (w454:bool[])
        n336 = Reverse 1D Array(array="Power Mon Chan Enable   \n  11    10      9      8       7       6      5       4       3       2      1       0") -> (reversed array=w408:bool[])
        n337 = Array Subset(array=w500, index=0, length=2) -> (w497:bool[])
        n338 = Array Subset(array=w495, index=0, length=2) -> (w334:bool[])
        n339 = Array Subset(array=w716, index=0, length=25) -> (w694:bool[])
        n340 = Reverse 1D Array(array="DIN Polarity \n  7      6        5      4       3       2      1       0") -> (reversed array=w407:bool[])
        n341 = Reverse 1D Array(array="Sync Input Polarity\n  2       1       0") -> (reversed array=w337:bool[])
        n342 = Array Subset(array=w636, index=0, length=3) -> (w627:bool[])
        n343 = Reverse 1D Array(array="DIN Demux Polarity\n  3       2       1      0") -> (reversed array=w335:bool[])
        n344 = Array Subset(array=w490, index=0, length=8) -> (w332:bool[])
        n345 = Build Array (concatenate)(w399, w712, w400, FALSE ("Read Register"), w712, w401, w712) -> (w523:bool[])
        n346 = Build Array (concatenate)(w708, w696, w696, w696, w696, w696) -> (w521:bool[])
        n347 = Build Array (concatenate)(w704, w695, w695, w695, w695, w695) -> (w542:bool[])
        n348 = Build Array (concatenate)(w402, w709, "User Reset", w710, w710, w710, w709, w709, w709) -> (w522:bool[])
        n349 = Number To Boolean Array(number="Power Mon Volt \nRef Threshold") -> (Boolean array=w385:bool[])
        n350 = Number To Boolean Array(number="DEMUX In Volt \nThreshold") -> (Boolean array=w371:bool[])
        n351 = Number To Boolean Array(number="DIN In Volt \nThreshold") -> (Boolean array=w357:bool[])
        n352 = Build Array (concatenate)(w454, w453, w452, w451, w450, w444, w443, w443) -> (w484:bool[])
        n353 = Number To Boolean Array(number="SYNC In \nVolt Threshold") -> (Boolean array=w343:bool[])
        n354 = Build Array (concatenate)(w699, FALSE ("Read Register"), w546, w546, w546, w546) -> (w520:bool[])
        n355 = Build Array (concatenate)(w647, w697, w697) -> (w519:bool[])
        n356 = Build Array (concatenate)(w408, bool[] [FALSE, FALSE, FALSE, FALSE] ("appended array"), w497, w333, w333, w334, w333, w333, w332) -> (w504:bool[])
        n357 = Build Array (concatenate)(w407, w690, w690, w337, w690, FALSE ("Read Register"), w335, w690) -> (w516:bool[])
        n358 = Boolean Array To Number(Boolean array=w521) -> (number=w537:u32)
        n359 = Boolean Array To Number(Boolean array=w523) -> (number=w541:u32)
        n360 = Boolean Array To Number(Boolean array=w522) -> (number=w539:u32)
        n361 = Build Array (concatenate)("Channel \nHold Order", "Channel \nTransfer Order", w630, w625, w625, w625, w627, w626, w625, w625, w625, w512, "SoftDEMUX \nSelector Enable", "Channel DEMUX \nSelector", w513) -> (w518:bool[])
        n362 = Build Array (concatenate)(w694, bool[] [FALSE, FALSE, FALSE, FALSE] ("appended array"), w692, w692, "Time Reset") -> (w517:bool[])
        n363 = Boolean Array To Number(Boolean array=w484) -> (number=w486:u32)
        n364 = Boolean Array To Number(Boolean array=w520) -> (number=w535:u32)
        n365 = Array Subset(array=w385, index=0, length=16) -> (w383:bool[])
        n366 = Array Subset(array=w371, index=0, length=16) -> (w369:bool[])
        n367 = Array Subset(array=w357, index=0, length=16) -> (w355:bool[])
        n368 = Array Subset(array=w343, index=0, length=16) -> (w341:bool[])
        n369 = Boolean Array To Number(Boolean array=w542) -> (number=w544:u32)
        n370 = Boolean Array To Number(Boolean array=w519) -> (number=w533:u32)
        n371 = Number To Hexadecimal String(1:i16 8 ("width (-)"), 2:w537) -> (0:w418:string)
        n372 = Boolean Array To Number(Boolean array=w504) -> (number=w506:u32)
        n373 = Number To Hexadecimal String(1:i16 8 ("width (-)"), 2:w541) -> (0:w411:string)
        n374 = Number To Hexadecimal String(1:i16 8 ("width (-)"), 2:w539) -> (0:w415:string)
        n375 = Boolean Array To Number(Boolean array=w516) -> (number=w527:u32)
        n376 = Number To Hexadecimal String(1:i16 8 ("width (-)"), 2:w486) -> (0:w481:string)
        n377 = Number To Hexadecimal String(1:i16 8 ("width (-)"), 2:w535) -> (0:w422:string)
        n378 = Boolean Array To Number(Boolean array=w517) -> (number=w529:u32)
        n379 = case shown="True" "Reset Register Map to Defaults" {
          tunnel: w338 -> [_ w842]
          tunnel: w339 -> [_ w841]
          tunnel: w514 -> [_ w847]
          frame False {
          }
          frame True {
            n380 = String To Byte Array(string=w847) -> (unsigned byte array=w846:u8[])
            n381 = Array Size(array=w846) -> (size(s)=w844:i32)
            n382 = Divide(x=w844, y=4) -> (x/y=w845:dbl)
            n383 = flat-sequence {
              tunnel: w842 -> [w851]
              tunnel: w841 -> [w850]
              tunnel: w847 -> [w849]
              tunnel: w845 -> [w848]
              tunnel: w842 -> [w862]
              tunnel: w841 -> [w861]
              tunnel: "r0000000000" ("data in") -> [w860]
              frame #0 {
                n384 = for {
                  N: w848 -> [_]
                  tunnel: w851 -> [w855]
                  tunnel: w850 -> [w854]
                  tunnel: w849 -> [w853]
                  i -> [w852]
                  n385 = call "RegisterMap2HexString.vi"("Word Num"=w852, "string"=w853) -> ("concatenated string"=w856:string)  [unwired: 9 in]
                  n386 = case shown="No Error" w854 {
                    tunnel: w855 -> [w859 _]
                    tunnel: w854 -> [w858 _]
                    tunnel: w856 -> [w857 _]
                    frame No Error {
                      n387 = Enqueue Element(queue=w859, element=w857, error in (no error)=w858) -> ()  [unwired: 1 in, 3 out]
                    }
                    frame Error {
                    }
                  }
                }
              }
              frame #1 {
                n388 = case shown="No Error" w861 {
                  tunnel: w861 -> [w865 _]
                  tunnel: w860 -> [w864 _]
                  tunnel: w862 -> [w863 _]
                  frame No Error {
                    n389 = Enqueue Element(queue=w863, element=w864, error in (no error)=w865) -> ()  [unwired: 1 in, 3 out]
                  }
                  frame Error {
                  }
                }
              }
            }
          }
        }
        n390 = Number To Hexadecimal String(1:i16 8 ("width (-)"), 2:w544) -> (0:w420:string)
        n391 = Number To Hexadecimal String(1:i16 8 ("width (-)"), 2:w533) -> (0:w427:string)
        n392 = Boolean Array To Number(Boolean array=w518) -> (number=w531:u32)
        n393 = Build Array (concatenate)(w383, w382, w382, w382, w382) -> (w392:bool[])
        n394 = Build Array (concatenate)(w369, w368, w368, w368, w368) -> (w378:bool[])
        n395 = Build Array (concatenate)(w355, w354, w354, w354, w354) -> (w364:bool[])
        n396 = Build Array (concatenate)(w341, w340, w340, w340, w340) -> (w350:bool[])
        n397 = Number To Hexadecimal String(1:i16 8 ("width (-)"), 2:w506) -> (0:w437:string)
        n398 = Number To Hexadecimal String(1:i16 8 ("width (-)"), 2:w527) -> (0:w435:string)
        n399 = Number To Hexadecimal String(1:i16 8 ("width (-)"), 2:w529) -> (0:w433:string)
        n400 = Number To Hexadecimal String(1:i16 8 ("width (-)"), 2:w531) -> (0:w430:string)
        n401 = local read "word2"() -> (w416:string)
        n402 = Boolean Array To Number(Boolean array=w392) -> (number=w394:u32)
        n403 = Boolean Array To Number(Boolean array=w378) -> (number=w380:u32)
        n404 = local read "wordA"() -> (w442:string)
        n405 = Boolean Array To Number(Boolean array=w364) -> (number=w366:u32)
        n406 = Boolean Array To Number(Boolean array=w350) -> (number=w352:u32)
        n407 = local read "word0"() -> (w410:string)
        n408 = local read "word1"() -> (w414:string)
        n409 = local read "wordB"() -> (w483:string)
        n410 = local read "word3"() -> (w419:string)
        n411 = local read "word5"() -> (w426:string)
        n412 = local read "word4"() -> (w423:string)
        n413 = local read "word9"() -> (w439:string)
        n414 = local read "word6"() -> (w428:string)
        n415 = local read "word8"() -> (w436:string)
        n416 = Number To Hexadecimal String(1:i16 8 ("width (-)"), 2:w394) -> (0:w389:string)
        n417 = Number To Hexadecimal String(1:i16 8 ("width (-)"), 2:w380) -> (0:w375:string)
        n418 = local read "word7"() -> (w432:string)
        n419 = Number To Hexadecimal String(1:i16 8 ("width (-)"), 2:w366) -> (0:w361:string)
        n420 = Number To Hexadecimal String(1:i16 8 ("width (-)"), 2:w352) -> (0:w347:string)
        n421 = Concatenate Strings("w00" ("string"), w411) -> (w664:string)
        n422 = Concatenate Strings("w02" ("string"), w418) -> (w653:string)
        n423 = Not Equal?(x=w441, y=w442) -> (x != y?=w440:bool)
        n424 = Concatenate Strings("w01" ("string"), w415) -> (w654:string)
        n425 = Not Equal?(x=w415, y=w414) -> (x != y?=w413:bool)
        n426 = Not Equal?(x=w411, y=w410) -> (x != y?=w412:bool)
        n427 = Not Equal?(x=w418, y=w416) -> (x != y?=w417:bool)
        n428 = local read "word30"() -> (w391:string)
        n429 = local read "word31"() -> (w377:string)
        n430 = local read "word32"() -> (w363:string)
        n431 = local read "word33"() -> (w349:string)
        n432 = Concatenate Strings("w05" ("string"), w427) -> (w651:string)
        n433 = Concatenate Strings("w03" ("string"), w420) -> (w545:string)
        n434 = Not Equal?(x=w420, y=w419) -> (x != y?=w421:bool)
        n435 = Concatenate Strings("w04" ("string"), w422) -> (w652:string)
        n436 = Not Equal?(x=w481, y=w483) -> (x != y?=w480:bool)
        n437 = Not Equal?(x=w422, y=w423) -> (x != y?=w424:bool)
        n438 = Not Equal?(x=w427, y=w426) -> (x != y?=w425:bool)
        n439 = Concatenate Strings("w09" ("string"), w437) -> (w507:string)
        n440 = Not Equal?(x=w437, y=w439) -> (x != y?=w438:bool)
        n441 = Not Equal?(x=w430, y=w428) -> (x != y?=w429:bool)
        n442 = Concatenate Strings("w0B" ("string"), w481) -> (w482:string)
        n443 = Not Equal?(x=w435, y=w436) -> (x != y?=w434:bool)
        n444 = Not Equal?(x=w433, y=w432) -> (x != y?=w431:bool)
        n445 = Concatenate Strings("w06" ("string"), w430) -> (w650:string)
        n446 = Concatenate Strings("w0A" ("string"), w441) -> (w509:string)
        n447 = Concatenate Strings("w07" ("string"), w433) -> (w649:string)
        n448 = Concatenate Strings("w08" ("string"), w435) -> (w648:string)
        n449 = Concatenate Strings("w30" ("string"), w389) -> (w390:string)
        n450 = Concatenate Strings("w31" ("string"), w375) -> (w376:string)
        n451 = Concatenate Strings("w32" ("string"), w361) -> (w362:string)
        n452 = Concatenate Strings("w33" ("string"), w347) -> (w348:string)
        n453 = Not Equal?(x=w389, y=w391) -> (x != y?=w388:bool)
        n454 = Not Equal?(x=w375, y=w377) -> (x != y?=w374:bool)
        n455 = Not Equal?(x=w361, y=w363) -> (x != y?=w360:bool)
        n456 = Not Equal?(x=w347, y=w349) -> (x != y?=w346:bool)
        n457 = case shown="True" w413 {
          tunnel: w654 -> [_ w829]
          tunnel: w338 -> [_ w827]
          tunnel: w339 -> [_ w828]
          tunnel: w415 -> [_ w826]
          frame False {
          }
          frame True {
            n458 = case shown="No Error" w828 {
              tunnel: w829 -> [w832 _]
              tunnel: w828 -> [w831 _]
              tunnel: w827 -> [w830 _]
              frame No Error {
                n459 = Enqueue Element(queue=w830, element=w832, error in (no error)=w831) -> ()  [unwired: 1 in, 3 out]
              }
              frame Error {
              }
            }
            "word1" <- w826
          }
        }
        n460 = case shown="True" w412 {
          tunnel: w664 -> [_ w836]
          tunnel: w338 -> [_ w835]
          tunnel: w339 -> [_ w834]
          tunnel: w411 -> [_ w833]
          frame False {
          }
          frame True {
            n461 = case shown="No Error" w834 {
              tunnel: w836 -> [w839 _]
              tunnel: w834 -> [w838 _]
              tunnel: w835 -> [w837 _]
              frame No Error {
                n462 = Enqueue Element(queue=w837, element=w839, error in (no error)=w838) -> ()  [unwired: 1 in, 3 out]
              }
              frame Error {
              }
            }
            "word0" <- w833
          }
        }
        n463 = case shown="True" w417 {
          tunnel: w653 -> [_ w822]
          tunnel: w338 -> [_ w821]
          tunnel: w339 -> [_ w820]
          tunnel: w418 -> [_ w819]
          frame False {
          }
          frame True {
            n464 = case shown="No Error" w820 {
              tunnel: w822 -> [w825 _]
              tunnel: w820 -> [w824 _]
              tunnel: w821 -> [w823 _]
              frame No Error {
                n465 = Enqueue Element(queue=w823, element=w825, error in (no error)=w824) -> ()  [unwired: 1 in, 3 out]
              }
              frame Error {
              }
            }
            "word2" <- w819
          }
        }
        n466 = case shown="True" w421 {
          tunnel: w545 -> [_ w815]
          tunnel: w338 -> [_ w814]
          tunnel: w339 -> [_ w813]
          tunnel: w420 -> [_ w812]
          frame False {
          }
          frame True {
            n467 = case shown="No Error" w813 {
              tunnel: w815 -> [w818 _]
              tunnel: w813 -> [w817 _]
              tunnel: w814 -> [w816 _]
              frame No Error {
                n468 = Enqueue Element(queue=w816, element=w818, error in (no error)=w817) -> ()  [unwired: 1 in, 3 out]
              }
              frame Error {
              }
            }
            "word3" <- w812
          }
        }
        n469 = case shown="True" w424 {
          tunnel: w652 -> [_ w808]
          tunnel: w338 -> [_ w807]
          tunnel: w339 -> [_ w806]
          tunnel: w422 -> [_ w805]
          frame False {
          }
          frame True {
            n470 = case shown="No Error" w806 {
              tunnel: w808 -> [w811 _]
              tunnel: w806 -> [w810 _]
              tunnel: w807 -> [w809 _]
              frame No Error {
                n471 = Enqueue Element(queue=w809, element=w811, error in (no error)=w810) -> ()  [unwired: 1 in, 3 out]
              }
              frame Error {
              }
            }
            "word4" <- w805
          }
        }
        n472 = case shown="True" w425 {
          tunnel: w651 -> [_ w801]
          tunnel: w338 -> [_ w800]
          tunnel: w339 -> [_ w799]
          tunnel: w427 -> [_ w798]
          frame False {
          }
          frame True {
            n473 = case shown="No Error" w799 {
              tunnel: w801 -> [w804 _]
              tunnel: w799 -> [w803 _]
              tunnel: w800 -> [w802 _]
              frame No Error {
                n474 = Enqueue Element(queue=w802, element=w804, error in (no error)=w803) -> ()  [unwired: 1 in, 3 out]
              }
              frame Error {
              }
            }
            "word5" <- w798
          }
        }
        n475 = case shown="True" w429 {
          tunnel: w650 -> [_ w794]
          tunnel: w338 -> [_ w793]
          tunnel: w339 -> [_ w792]
          tunnel: w430 -> [_ w791]
          frame False {
          }
          frame True {
            n476 = case shown="No Error" w792 {
              tunnel: w794 -> [w797 _]
              tunnel: w792 -> [w796 _]
              tunnel: w793 -> [w795 _]
              frame No Error {
                n477 = Enqueue Element(queue=w795, element=w797, error in (no error)=w796) -> ()  [unwired: 1 in, 3 out]
              }
              frame Error {
              }
            }
            "word6" <- w791
          }
        }
        n478 = case shown="True" w431 {
          tunnel: w649 -> [_ w787]
          tunnel: w338 -> [_ w786]
          tunnel: w339 -> [_ w785]
          tunnel: w433 -> [_ w784]
          frame False {
          }
          frame True {
            n479 = case shown="No Error" w785 {
              tunnel: w787 -> [w790 _]
              tunnel: w785 -> [w789 _]
              tunnel: w786 -> [w788 _]
              frame No Error {
                n480 = Enqueue Element(queue=w788, element=w790, error in (no error)=w789) -> ()  [unwired: 1 in, 3 out]
              }
              frame Error {
              }
            }
            "word7" <- w784
          }
        }
        n481 = case shown="True" w434 {
          tunnel: w648 -> [_ w780]
          tunnel: w338 -> [_ w779]
          tunnel: w339 -> [_ w778]
          tunnel: w435 -> [_ w777]
          frame False {
          }
          frame True {
            n482 = case shown="No Error" w778 {
              tunnel: w780 -> [w783 _]
              tunnel: w778 -> [w782 _]
              tunnel: w779 -> [w781 _]
              frame No Error {
                n483 = Enqueue Element(queue=w781, element=w783, error in (no error)=w782) -> ()  [unwired: 1 in, 3 out]
              }
              frame Error {
              }
            }
            "word8" <- w777
          }
        }
        n484 = case shown="True" w438 {
          tunnel: w507 -> [_ w773]
          tunnel: w338 -> [_ w772]
          tunnel: w339 -> [_ w771]
          tunnel: w437 -> [_ w770]
          frame False {
          }
          frame True {
            n485 = case shown="No Error" w771 {
              tunnel: w773 -> [w776 _]
              tunnel: w771 -> [w775 _]
              tunnel: w772 -> [w774 _]
              frame No Error {
                n486 = Enqueue Element(queue=w774, element=w776, error in (no error)=w775) -> ()  [unwired: 1 in, 3 out]
              }
              frame Error {
              }
            }
            "word9" <- w770
          }
        }
        n487 = case shown="True" w440 {
          tunnel: w509 -> [_ w766]
          tunnel: w338 -> [_ w765]
          tunnel: w339 -> [_ w764]
          tunnel: w441 -> [_ w763]
          frame False {
          }
          frame True {
            n488 = case shown="No Error" w764 {
              tunnel: w766 -> [w769 _]
              tunnel: w764 -> [w768 _]
              tunnel: w765 -> [w767 _]
              frame No Error {
                n489 = Enqueue Element(queue=w767, element=w769, error in (no error)=w768) -> ()  [unwired: 1 in, 3 out]
              }
              frame Error {
              }
            }
            "wordA" <- w763
          }
        }
        n490 = case shown="True" w480 {
          tunnel: w482 -> [_ w759]
          tunnel: w338 -> [_ w758]
          tunnel: w339 -> [_ w757]
          tunnel: w481 -> [_ w756]
          frame False {
          }
          frame True {
            n491 = case shown="No Error" w757 {
              tunnel: w759 -> [w762 _]
              tunnel: w757 -> [w761 _]
              tunnel: w758 -> [w760 _]
              frame No Error {
                n492 = Enqueue Element(queue=w760, element=w762, error in (no error)=w761) -> ()  [unwired: 1 in, 3 out]
              }
              frame Error {
              }
            }
            "wordB" <- w756
          }
        }
        n493 = case shown="True" w388 {
          tunnel: w390 -> [_ w752]
          tunnel: w338 -> [_ w751]
          tunnel: w339 -> [_ w750]
          tunnel: w389 -> [_ w749]
          frame False {
          }
          frame True {
            n494 = case shown="No Error" w750 {
              tunnel: w752 -> [w755 _]
              tunnel: w750 -> [w754 _]
              tunnel: w751 -> [w753 _]
              frame No Error {
                n495 = Enqueue Element(queue=w753, element=w755, error in (no error)=w754) -> ()  [unwired: 1 in, 3 out]
              }
              frame Error {
              }
            }
            "word30" <- w749
          }
        }
        n496 = case shown="True" w374 {
          tunnel: w376 -> [_ w745]
          tunnel: w338 -> [_ w744]
          tunnel: w339 -> [_ w743]
          tunnel: w375 -> [_ w742]
          frame False {
          }
          frame True {
            n497 = case shown="No Error" w743 {
              tunnel: w745 -> [w748 _]
              tunnel: w743 -> [w747 _]
              tunnel: w744 -> [w746 _]
              frame No Error {
                n498 = Enqueue Element(queue=w746, element=w748, error in (no error)=w747) -> ()  [unwired: 1 in, 3 out]
              }
              frame Error {
              }
            }
            "word31" <- w742
          }
        }
        n499 = case shown="True" w360 {
          tunnel: w362 -> [_ w738]
          tunnel: w338 -> [_ w737]
          tunnel: w339 -> [_ w736]
          tunnel: w361 -> [_ w735]
          frame False {
          }
          frame True {
            n500 = case shown="No Error" w736 {
              tunnel: w738 -> [w741 _]
              tunnel: w736 -> [w740 _]
              tunnel: w737 -> [w739 _]
              frame No Error {
                n501 = Enqueue Element(queue=w739, element=w741, error in (no error)=w740) -> ()  [unwired: 1 in, 3 out]
              }
              frame Error {
              }
            }
            "word32" <- w735
          }
        }
        n502 = case shown="True" w346 {
          tunnel: w348 -> [_ w731]
          tunnel: w338 -> [_ w730]
          tunnel: w339 -> [_ w729]
          tunnel: w347 -> [_ w728]
          frame False {
          }
          frame True {
            n503 = case shown="No Error" w729 {
              tunnel: w731 -> [w734 _]
              tunnel: w729 -> [w733 _]
              tunnel: w730 -> [w732 _]
              frame No Error {
                n504 = Enqueue Element(queue=w732, element=w734, error in (no error)=w733) -> ()  [unwired: 1 in, 3 out]
              }
              frame Error {
              }
            }
            "word33" <- w728
          }
        }
      }
    }
  }
